vi "GE 5565PIORC.PIO.Write (1D U32).vi"(7 "byte order (big-endian)":T1(ring), 8 "error in (no error)":errorcluster, 9 "data":u32[](array[numeric]), 10 "offset":u32, 11 "GE 5565PIORC in":refnum<class "GE 5565PIORC.lvclass">) -> (0 "error out":errorcluster, 1 "data out":u32[](array[numeric]), 3 "GE 5565PIORC out":refnum<class "GE 5565PIORC.lvclass">)   [LabVIEW 2020, in "GE 5565PIORC.lvclass"]
doc: "Writes the contents of <B>data</B> to the specified <B>offset</B>. The number of elements transferred will be the number of elements in <B>data</B>."
uses:
  GE 5565PIORC.lvclass
  <vilib>/Instr/_visa.llb/VISA Register Access Address Space.ctl
  GE 5565PIORC.lvclass/GE 5565PIORC.ctl
  GE 5565PIORC.VISA.Move Out.String (U8).vi
  GE 5565PIORC.VISA.Return Handler.vi
  <vilib>/Utility/error.llb/Error Cluster From Error Code.vi
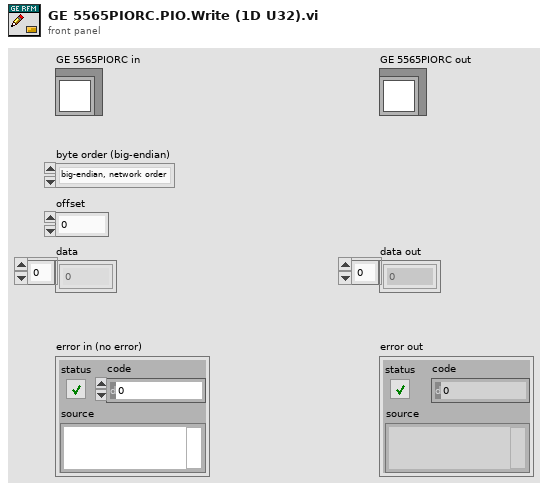
[diagram p1: front panel]
types:
  T1 = enum16{"big-endian, network order", "native, host order", "little-endian"}
  T2 = typedef "VISA Register Access Address Space.ctl" = u16
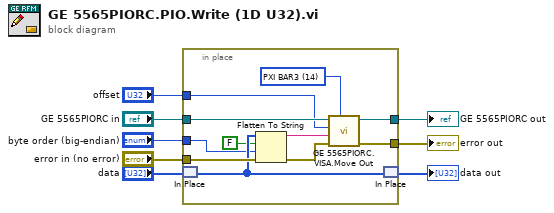
[diagram p0: block diagram]
diagram:
  n1 = in-place {
    in-place-border: "error in (no error)" -> [w17]
    in-place-border: [w15] -> w7
    in-place-border: "GE 5565PIORC in" -> [w18]
    in-place-border: "offset" -> [w13]
    in-place-border: "byte order (big-endian)" -> [w9]
    in-place-border: [w12] -> w1
    w19 = T2 14 items=["VXI/VME A16"=1, "VXI/VME A24"=2, "VXI/VME A32"=3, "VXI/VME A64"=4, "PXI Memory Allocations"=9, "PXI Configuration"=10, "PXI BAR0"=11, "PXI BAR1"=12, "PXI BAR2"=13, "PXI BAR3"=14, "PXI BAR4"=15, "PXI BAR5"=16] ("address space")
    n2 = in-place-match #1("data") -> (w11:u32[])
    n3 = Flatten To String(anything=w11, prepend array or string size? (T)=FALSE, byte order (0:big-endian, network order)=w9, error in (no error)=w17) -> (data string=w14:string, error out=w16:errorcluster)  [unwired: 1 out]
    n4 = call-poly "GE 5565PIORC.VISA.Move Out.vi"("address space"=w19, "error in (no error)"=w16, "data in"=w14, "offset"=w13, "GE 5565PIORC in"=w18) -> ("error out"=w15:errorcluster, "GE 5565PIORC out"=w12:refnum<class "GE 5565PIORC.lvclass">)  [unwired: 4 in, 1 out]
    n5 = in-place-match #1(w11) -> (→"data out":u32[])
  }
  "GE 5565PIORC out" <- w1
  "error out" <- w7
